vi "NTJ_Convert String to NT String Array Buffer.vi"(11 "LV Buffer":string) -> (3 "NT Buffer":string)   [LabVIEW 2019]
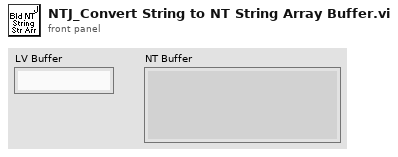
[diagram p1: front panel]
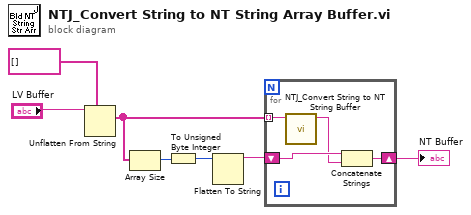
[diagram p0: block diagram]
diagram:
  n1 = Unflatten From String(type=string[] [], binary string="LV Buffer") -> (value=w5:string[])  [unwired: 3 in, 2 out]
  n2 = Array Size(array=w5) -> (size(s)=w4:i32)
  n3 = To Unsigned Byte Integer(number=w4) -> (unsigned 8bit integer=w3:u8)
  n4 = Flatten To String(anything=w3) -> (data string=w2:string)  [unwired: 3 in, 2 out]
  n5 = for {
    tunnel: w5 -> [w11] mode=indexing
    shift-right: [w9] -> w1
    shift-left: w2 -> [w10]
    n6 = call "NTJ_Convert String to NT String Buffer.vi"("LV Buffer"=w11) -> ("NT Buffer"=w8:string)  [unwired: 10 in]
    n7 = Concatenate Strings(w10, w8) -> (w9:string)
  }
  "NT Buffer" <- w1
